vi "Chase Host.vi"() -> ()   [LabVIEW 2012]
panel:
  out "Image 2":T1(plugin-control)
  out "Image":T1(plugin-control)
  out "Matches (Color Pattern Matching 1)":T2(array[cluster]) {"Bounding Box"."y" format="%.2f"; "Bounding Box"."x" format="%.2f"; "Position"."y" format="%.2f"; "Position"."x" format="%.2f"; "Score" format="%.2f"; "Scale" format="%.2f"; "Angle" format="%.2f"}
  out "Matches (Color Location 1)":T2(array[cluster]) {"Bounding Box"."y" format="%.2f"; "Bounding Box"."x" format="%.2f"; "Position"."y" format="%.2f"; "Position"."x" format="%.2f"; "Score" format="%.2f"; "Scale" format="%.2f"; "Angle" format="%.2f"}
  in  "stop":bool
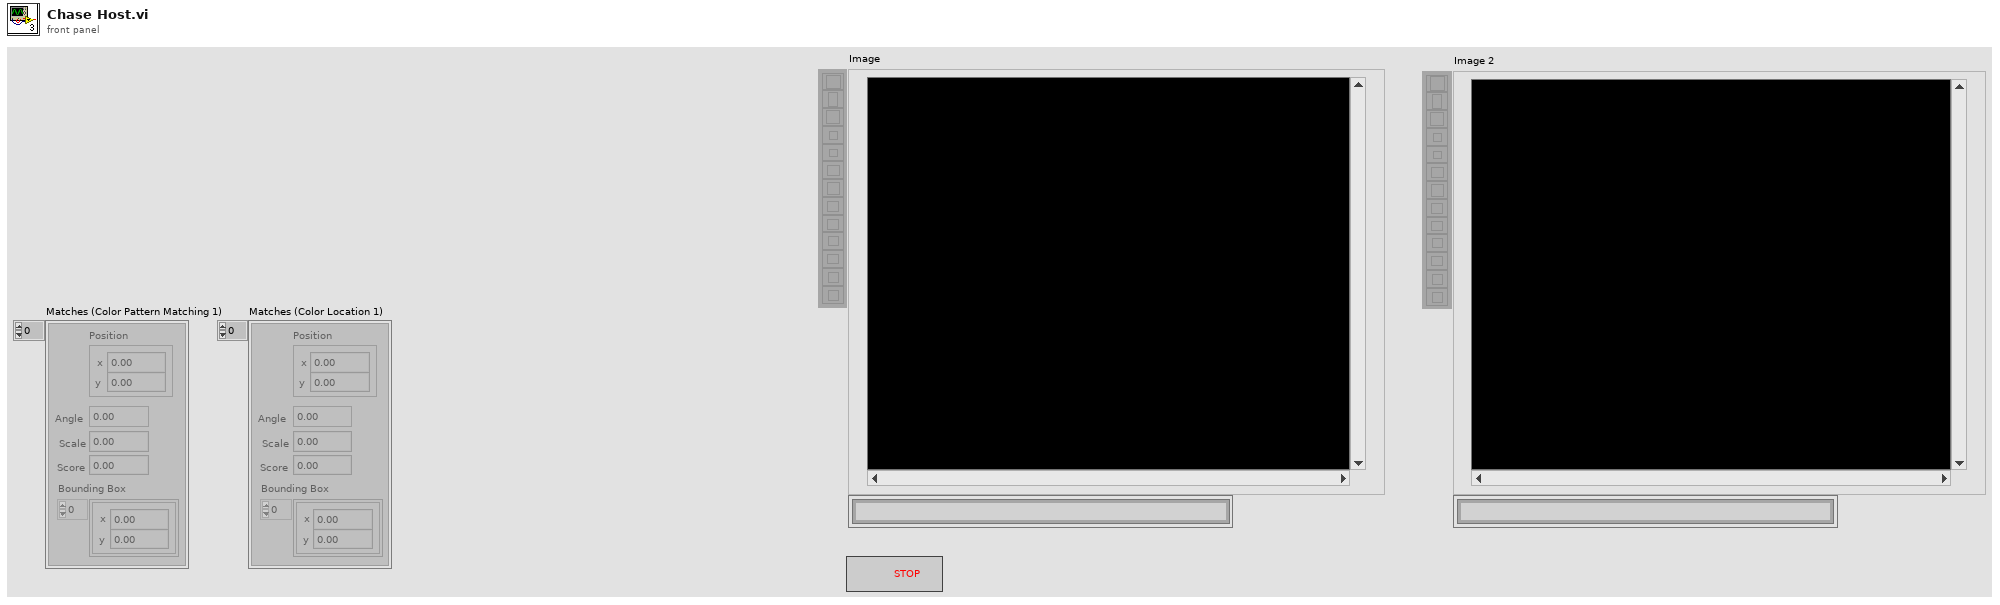
[diagram p1: front panel]
types:
  T1 = typedef "IMAQ Image.ctl" = refnum<image>
  T2 = cluster{"Position":cluster{"x":sgl, "y":sgl}, "Angle":sgl, "Scale":sgl, "Score":sgl, "Bounding Box":cluster{"x":sgl, "y":sgl}[]}[]
  T3 = cluster{"Global Rectangle":cluster{"x1Left":i32, "y1Top":i32, "x2Right":i32, "y2Bottom":i32}, "Centroid":cluster{"x":sgl, "y":sgl}, "Object Size":u32, "Score":dbl}[]
  T4 = cluster{"Shape Report (Shape Matching 1)[0]":cluster{"Global Rectangle":cluster{"x1Left":i32, "y1Top":i32, "x2Right":i32, "y2Bottom":i32}, "Centroid":cluster{"x":sgl, "y":sgl}, "Object Size":u32, "Score":dbl}, "Shape Report (Shape Matching 1)[1]":cluster{"Global Rectangle":cluster{"x1Left":i32, "y1Top":i32, "x2Right":i32, "y2Bottom":i32}, "Centroid":cluster{"x":sgl, "y":sgl}, "Object Size":u32, "Score":dbl}, "Shape Report (Shape Matching 1)[2]":cluster{"Global Rectangle":cluster{"x1Left":i32, "y1Top":i32, "x2Right":i32, "y2Bottom":i32}, "Centroid":cluster{"x":sgl, "y":sgl}, "Object Size":u32, "Score":dbl}, "Shape Report (Shape Matching 1)[3]":cluster{"Global Rectangle":cluster{"x1Left":i32, "y1Top":i32, "x2Right":i32, "y2Bottom":i32}, "Centroid":cluster{"x":sgl, "y":sgl}, "Object Size":u32, "Score":dbl}, "Shape Report (Shape Matching 1)[4]":cluster{"Global Rectangle":cluster{"x1Left":i32, "y1Top":i32, "x2Right":i32, "y2Bottom":i32}, "Centroid":cluster{"x":sgl, "y":sgl}, "Object Size":u32, "Score":dbl}, "Shape Report (Shape Matching 1)[5]":cluster{"Global Rectangle":cluster{"x1Left":i32, "y1Top":i32, "x2Right":i32, "y2Bottom":i32}, "Centroid":cluster{"x":sgl, "y":sgl}, "Object Size":u32, "Score":dbl}, "Shape Report (Shape Matching 1)[6]":cluster{"Global Rectangle":cluster{"x1Left":i32, "y1Top":i32, "x2Right":i32, "y2Bottom":i32}, "Centroid":cluster{"x":sgl, "y":sgl}, "Object Size":u32, "Score":dbl}, "Shape Report (Shape Matching 1)[7]":cluster{"Global Rectangle":cluster{"x1Left":i32, "y1Top":i32, "x2Right":i32, "y2Bottom":i32}, "Centroid":cluster{"x":sgl, "y":sgl}, "Object Size":u32, "Score":dbl}, "Shape Report (Shape Matching 1)[8]":cluster{"Global Rectangle":cluster{"x1Left":i32, "y1Top":i32, "x2Right":i32, "y2Bottom":i32}, "Centroid":cluster{"x":sgl, "y":sgl}, "Object Size":u32, "Score":dbl}}
  T5 = cluster{"x1Left":i32, "y1Top":i32, "x2Right":i32, "y2Bottom":i32}
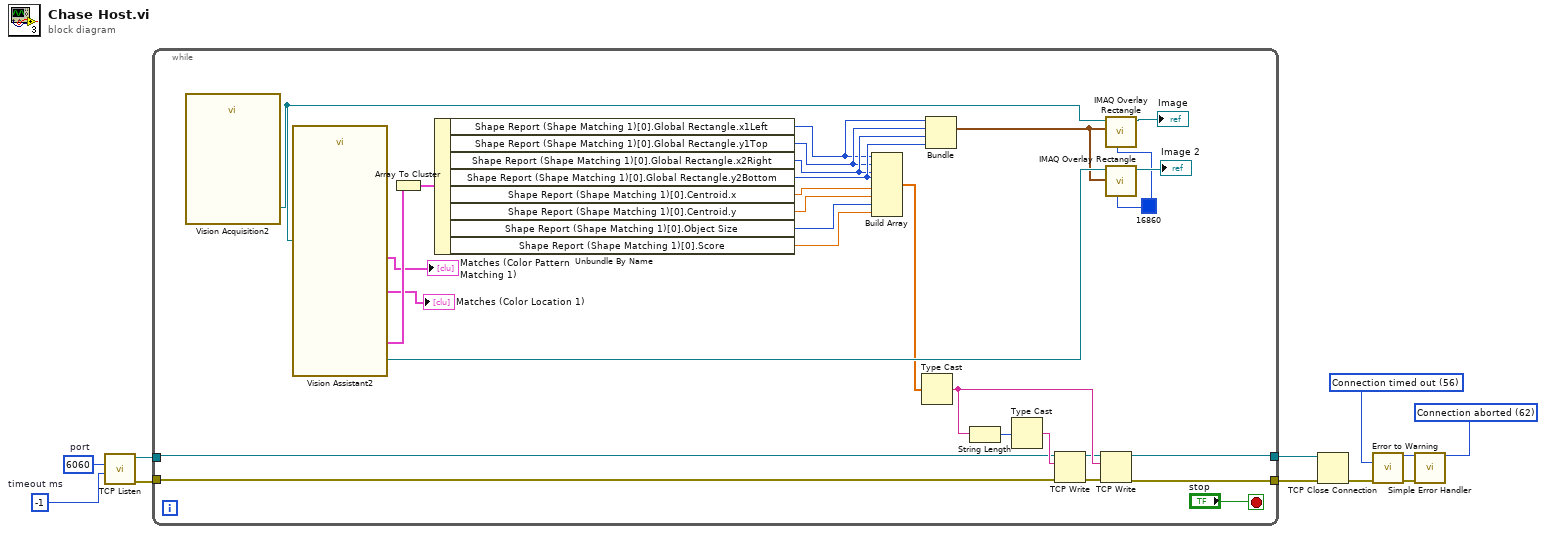
[diagram p0: block diagram]
diagram:
  w4 = 56 items=["No Error", "Argument Error", "Memory Full", "Out of Zone", "End of File", "File Already Open", "Generic File IO Error", "File Not Found", "File Permission Error", "Disk Full", "Duplicate Path", "Too Many Files Open", "Not Enabled", "Resource File Not Found", "Cannot Add Resource", "Resource Not Found", "Image Not Found", "Image Memory Error", "Pen Does Not Exist", "Config Bad Type", "Config Token Not Found", "Config Parse Error", "Config Memory Error", "Bad External Code Format", "Bad External Code Offset", "External Code Not Present", "Null Window", "Destroy Window Mixup", "Null Menu", "Print Aborted", "Bad Print Record", "Print Driver Error", "Windows Error During Print", "Memory Error During Print", "Print Dialog Error", "Generic Print Error", "Invalid Device Refnum", "Device Not Found", "Device Parameter Error", "Device Unit Error", "Can't Open Device", "Device Call Aborted", "Generic Error", "Cancelled By User", "Object ID Too Low", "Object ID Too High", "Object Not In Heap", "Unknown Heap", "Bad DefProc ID", "DefProc Not In Table", "Message Out Of Range", "Null Method", "Unknown Message", "Manager Call Not Supported", "Bad address", "Connection In progress", "Connection timed out", "Connection is already in progress", "Network attribute not supported", "Network error", "Address in use", "System out of memory", "Connection aborted", "Connection refused", "Connection is not connected", "Connection is already connected", "Connection closed", "Initialize error (interapplication manager)", "Bad occurrence", "Wait on unbound occurrence handler", "Occurrence queue overflow", "Bad path", "Semaphore not signaled", "Unrecognized type (interapplication manager)"] ("2nd Error to Convert")
  w5 = 62 items=["No Error", "Argument Error", "Memory Full", "Out of Zone", "End of File", "File Already Open", "Generic File IO Error", "File Not Found", "File Permission Error", "Disk Full", "Duplicate Path", "Too Many Files Open", "Not Enabled", "Resource File Not Found", "Cannot Add Resource", "Resource Not Found", "Image Not Found", "Image Memory Error", "Pen Does Not Exist", "Config Bad Type", "Config Token Not Found", "Config Parse Error", "Config Memory Error", "Bad External Code Format", "Bad External Code Offset", "External Code Not Present", "Null Window", "Destroy Window Mixup", "Null Menu", "Print Aborted", "Bad Print Record", "Print Driver Error", "Windows Error During Print", "Memory Error During Print", "Print Dialog Error", "Generic Print Error", "Invalid Device Refnum", "Device Not Found", "Device Parameter Error", "Device Unit Error", "Can't Open Device", "Device Call Aborted", "Generic Error", "Cancelled By User", "Object ID Too Low", "Object ID Too High", "Object Not In Heap", "Unknown Heap", "Bad DefProc ID", "DefProc Not In Table", "Message Out Of Range", "Null Method", "Unknown Message", "Manager Call Not Supported", "Bad address", "Connection In progress", "Connection timed out", "Connection is already in progress", "Network attribute not supported", "Network error", "Address in use", "System out of memory", "Connection aborted", "Connection refused", "Connection is not connected", "Connection is already connected", "Connection closed", "Initialize error (interapplication manager)", "Bad occurrence", "Wait on unbound occurrence handler", "Occurrence queue overflow", "Bad path", "Semaphore not signaled", "Unrecognized type (interapplication manager)"] ("1st Error to Convert")
  w9 = u16 6060  # port
  w10 = -1  # timeout ms
  n1 = call <vilib>:"TCP Listen.vi"("timeout ms (wait forever: -1)"=w10, "port"=w9) -> ("error out"=w1:errorcluster, "connection ID"=w8:refnum<k5>)  [unwired: 5 in, 3 out]
  n2 = while {
    tunnel: w8 -> [w33]
    tunnel: [w32] -> w3
    tunnel: [w31] -> w2
    tunnel: w1 -> [w30]
    stop <- "stop" stop-if-true
    w19 = u32 16860 ("Color")
    n3 = call "Vision Acquisition2"() -> ("Image Out"=w18:T1)  [unwired: 25 in, 2 out]
    n4 = call "Vision Assistant2"("Image In"=w18) -> ("Image Out"=w17:T1, "Shape Report (Shape Matching 1)"=w28:T3, "Matches (Color Pattern Matching 1)"=→"Matches (Color Pattern Matching 1)":T2, "Matches (Color Location 1)"=→"Matches (Color Location 1)":T2)  [unwired: 19 in, 4 out]
    n5 = Array To Cluster(array=w28) -> (cluster=w29:T4)
    n6 = Unbundle By Name(w29) -> ("Shape Report (Shape Matching 1)[0].Global Rectangle.x1Left"=w13:i32, "Shape Report (Shape Matching 1)[0].Global Rectangle.y1Top"=w14:i32, "Shape Report (Shape Matching 1)[0].Global Rectangle.x2Right"=w15:i32, "Shape Report (Shape Matching 1)[0].Global Rectangle.y2Bottom"=w16:i32, "Shape Report (Shape Matching 1)[0].Centroid.x"=w25:sgl, "Shape Report (Shape Matching 1)[0].Centroid.y"=w24:sgl, "Shape Report (Shape Matching 1)[0].Object Size"=w23:u32, "Shape Report (Shape Matching 1)[0].Score"=w22:dbl)
    n7 = Build Array(w13, w14, w15, w16, w25, w24, w23, w22) -> (w11:dbl[])
    n8 = Type Cast(x=w11) -> (*(type *) &x=w38:string)  [unwired: 1 in]
    n9 = Bundle("x1Left"=w13, "y1Top"=w14, "x2Right"=w15, "y2Bottom"=w16) -> (w12:T5)  [unwired: 1 in]
    n10 = String Length(string=w38) -> (length=w36:i32)
    n11 = Type Cast(x=w36) -> (*(type *) &x=w37:string)  [unwired: 1 in]
    n12 = TCP Write(connection ID=w33, data in=w37, error in (no error)=w30) -> (connection ID out=w34:refnum<k5>, error out=w35:errorcluster)  [unwired: 1 in, 1 out]
    n13 = TCP Write(connection ID=w34, data in=w38, error in (no error)=w35) -> (connection ID out=w32:refnum<k5>, error out=w31:errorcluster)  [unwired: 1 in, 1 out]
    n14 = call "IMAQ Overlay Rectangle"("Color"=w19, "Rectangle"=w12, "Image"=w18) -> ("Image Out"=→"Image":T1)  [unwired: 7 in, 1 out]
    n15 = call "IMAQ Overlay Rectangle"("Color"=w19, "Rectangle"=w12, "Image"=w17) -> ("Image Out"=→"Image 2":T1)  [unwired: 7 in, 1 out]
  }
  n16 = TCP Close Connection(connection ID=w3, error in (no error)=w2) -> (error out=w7:errorcluster)  [unwired: 1 in, 1 out]
  n17 = call <vilib>:"Error to Warning.vi"("1st Error to Convert"=w5, "2nd Error to Convert"=w4, "error in"=w7) -> ("warning out"=w6:errorcluster)  [unwired: 12 in]
  n18 = call <vilib>:"Simple Error Handler.vi"("error in (no error)"=w6) -> ()  [unwired: 4 in, 5 out]
